vi "Find Workspace.vi"(8 "Error In":errorcluster, 10 "Control In":T2, 11 "Carrier Tray in":refnum<class "Assembly Tray.lvclass">) -> (0 "Error Out":errorcluster, 1 "Workspace":T1, 2 "Control Out":T2, 3 "Carrier Tray Out":refnum<class "Assembly Tray.lvclass">)   [LabVIEW 2020, in "Assembly Tray.lvclass"]
uses:
  Assembly Tray.lvclass
  C:/Users/hep/Documents/CMU gantry/Classes/Workspace/Fixture.lvclass
  Controller/Controllers.ctl
  Controller/I-O/I-O.lvclass
  Controller/Dispenser/Dispenser.lvclass
  C:/Program Files (x86)/Aerotech/A3200/LabVIEW/2010/Bin/Aerotech.A3200.dll
  Program Files (x86)/Aerotech/A3200/LabVIEW/2010/Bin/Aerotech.A3200.dll
  Workspace.ctl
  Fixture.lvclass/Fixture.ctl
  Assembly Tray.lvclass/Assembly Tray.ctl
  Read Fixture ID.vi
  Fixture.lvclass
  Controller/Controller.lvclass
panel:
  in  "output cluster 2":T1
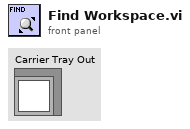
[diagram p1: front panel]
types:
  T1 = typedef "Fixture.lvclass/Workspace.ctl" = cluster{"XYZTheta":dbl[], "Workspace Valve":i32, "Workspace Sensor":i32}
  T2 = typedef "Controller.lvclass/Controllers.ctl" = cluster{"I-O.lvclass":refnum<class "I-O.lvclass">, "Dispenser.lvclass":refnum<class "Dispenser.lvclass">, "Gantry":refnum<k24>}
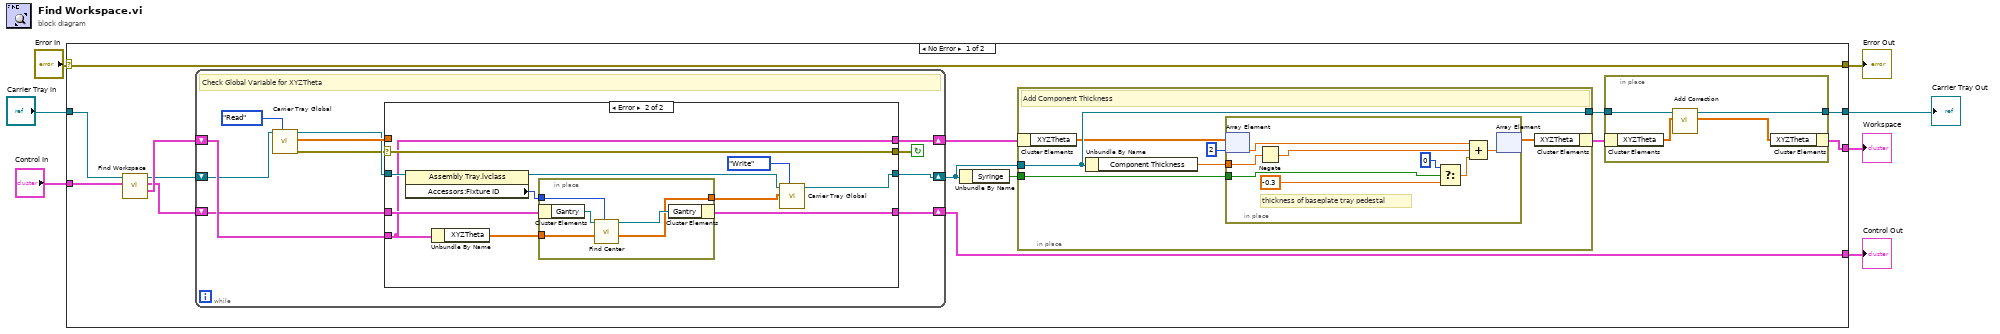
[diagram p0: block diagram]
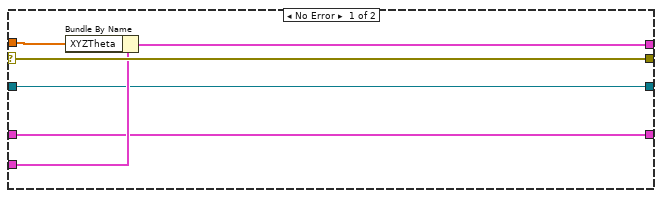
[diagram p2: hidden frame]
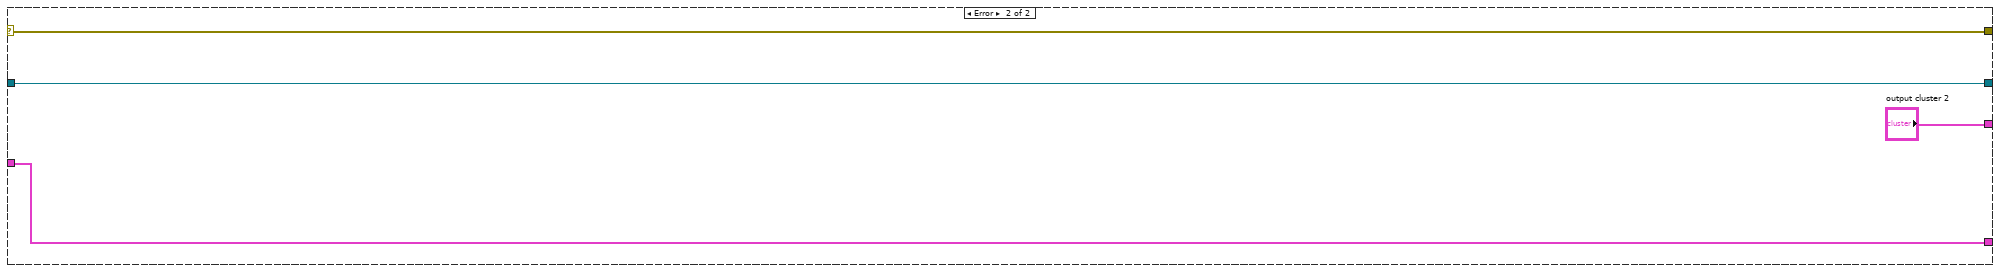
[diagram p3: hidden frame]
diagram:
  n1 = case shown="No Error" "Error In" {
    selector: "Error In" -> [w21 w75]
    tunnel: [w21 w75] -> w6
    tunnel: "Control In" -> [w20 w76]
    tunnel: [w16 w76] -> w4
    tunnel: "Carrier Tray in" -> [w19 w73]
    tunnel: [w17 "output cluster 2"] -> w2
    tunnel: [w18 w73] -> w1
    frame No Error {
      n2 = call-parent "Find Workspace.vi"("Control In"=w20, "Workspace In"=w19) -> (1:"Workspace Out"=w15:T1, "Control Out"=w14:T2, 3:"Workspace Out"=w8:refnum<class "Assembly Tray.lvclass">)  [unwired: 6 in, 1 out]
      n3 = while {
        shift-right: [w43] -> w13
        shift-left: w8 -> [w41]
        shift-right: [w45] -> w16
        shift-left: w14 -> [w46]
        shift-right: [w42] -> w12
        shift-left: w15 -> [w47]
        stop <- w49 continue-if-true
        # "Check Global Variable for XYZTheta"
        n4 = call "Carrier Tray Global.vi"("Action"=enum16{"Initialize", "Read", "Write"}."Read", "Carrier Tray.lvclass"=w41) -> ("error out"=w40:errorcluster, "XYZTheta out"=w48:dbl[], "Carrier Tray.lvclass 2"=w44:refnum<class "Assembly Tray.lvclass">)  [unwired: 7 in]
        n5 = case shown="Error" w40 {
          selector: w40 -> [w56 w67]
          tunnel: [w56 w67] -> w49
          tunnel: w48 -> [w55 _]
          tunnel: [w54 w57] -> w42
          tunnel: w47 -> [w53 w57]
          tunnel: w46 -> [w51 w61]
          tunnel: [w51 w60] -> w45
          tunnel: w44 -> [w52 w64]
          tunnel: [w52 w66] -> w43
          frame No Error {
            n6 = Bundle By Name(cluster=w53, "XYZTheta"=w55) -> (w54:T1)
          }
          frame Error {
            n7 = property class="Assembly Tray.lvclass"(reference=w64) -> (reference out=w63:refnum<class "Assembly Tray.lvclass">, "Accessors:Fixture ID"=w62:i32)  [unwired: 1 in, 1 out]
            n8 = Unbundle By Name(w57) -> ("XYZTheta"=w59:dbl[])
            n9 = in-place {
              in-place-border: w62 -> [w72]
              in-place-border: w59 -> [w69]
              in-place-border: [w68] -> w58
              n10 = in-place-cluster #1(w61) -> ("Gantry"=w71:refnum<k24>)
              n11 = call "Find Center.vi"("Tray Number"=w72, "XYZTheta"=w69, "Gantry 2"=w71) -> ("XYZTheta Centers"=w68:dbl[][], "Gantry 3"=w70:refnum<k24>)  [unwired: 7 in]
              n12 = in-place-cluster #1("Gantry"=w70) -> (w60:T2)
            }
            n13 = call "Carrier Tray Global.vi"("Action"=enum16{"Initialize", "Read", "Write"}."Write", "XYZTheta in"=w58, "Carrier Tray.lvclass"=w63) -> ("Carrier Tray.lvclass 2"=w66:refnum<class "Assembly Tray.lvclass">)  [unwired: 6 in, 2 out]
          }
        }
      }
      n14 = Unbundle By Name(w13) -> ("Syringe"=w11:bool)
      n15 = in-place {
        in-place-border: w13 -> [w24]
        in-place-border: [w24] -> w10
        in-place-border: w11 -> [w23]
        # "Add Component Thickness"
        n16 = in-place-cluster #2(w12) -> ("XYZTheta"=w22:dbl[])
        n17 = Unbundle By Name(w24) -> ("Component Thickness"=w25:dbl)
        n18 = in-place {
          in-place-border: w25 -> [w29]
          in-place-border: w23 -> [w34]
          # "thickness of baseplate tray pedestal"
          n19 = in-place-array #3(w22, 2) -> (w30:dbl)
          n20 = Negate(x=w29) -> (-x=w28:dbl)
          n21 = Select(t=0, s=w34, f=-0.3) -> (s? t:f=w31:dbl)
          n22 = Compound Arithmetic op=ADD(w30, w28, w31) -> (w35:dbl)
          n23 = in-place-array #3(w35) -> (w26:dbl[])  [unwired: 1 out]
        }
        n24 = in-place-cluster #2("XYZTheta"=w26) -> (w9:T1)
      }
      n25 = in-place {
        in-place-border: [w39] -> w18
        in-place-border: w10 -> [w38]
        n26 = in-place-cluster #4(w9) -> ("XYZTheta"=w37:dbl[])
        n27 = call "Add Correction.vi"("XYZTheta"=w37, "Carrier Tray in"=w38) -> ("XYZTheta Out"=w36:dbl[], "Carrier Tray out"=w39:refnum<class "Assembly Tray.lvclass">)  [unwired: 7 in, 1 out]
        n28 = in-place-cluster #4("XYZTheta"=w36) -> (w17:T1)
      }
    }
    frame Error {
    }
  }
  "Error Out" <- w6
  "Control Out" <- w4
  "Workspace" <- w2
  "Carrier Tray Out" <- w1
